vi "ADCP过程数据编码.vi"() -> (3 "发送的信息":string)   [LabVIEW 2016, in "数据传输系统-03.lvlib"]
panel:
  out "数值":i32
  out "层数":string
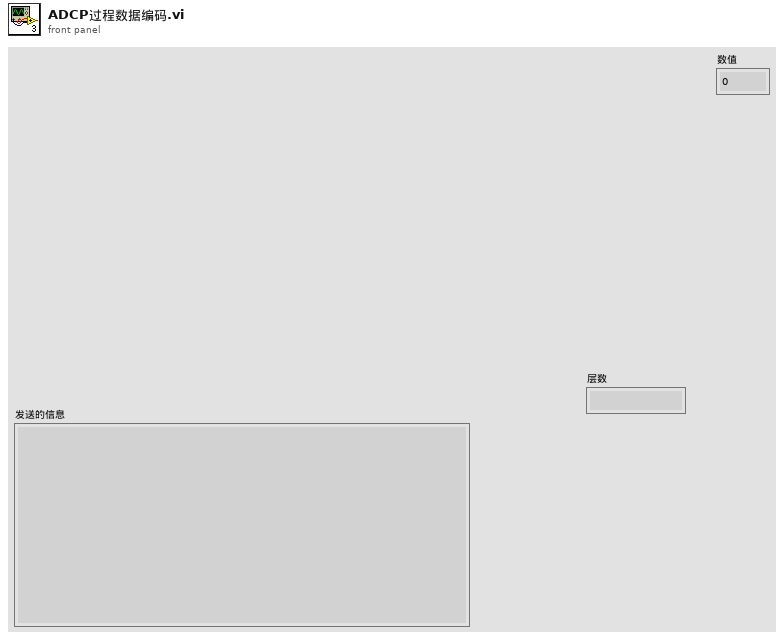
[diagram p1: front panel]
types:
  T1 = cluster{"CODMn":string, "CODCr":string, "DO":string, "铜":string, "PH":string, "氨氮":string, "比电导率":string, "水温":string, "COD":string, "浊度":string, "总氮":string, "总磷":string, "叶绿素a":string, "藻密度":string, "水位":string, "流速":string, "方向":string, "瞬时流量":string, "累积流量":string, "正累积流量":string, "负累积流量":string, "亚硝酸盐":string, "硫化物":string, "ORP":string, "铅":string, "镉":string, "锌":string, "镍":string, "锰":string, "汞":string, "气温":string, "气压":string, "风速":string, "风向":string, "空气温度":string, "相对湿度":string, "分钟雨量":string, "小时雨量":string, "日雨量":string, "累积雨量":string, "盐度":string, "磷酸盐":string, "硝氮":string, "氟化物":string, "挥发酚":string, "氯化物":string, "蓝绿藻":string, "余氯":string, "综合生物毒性":string, "艏向":string, "横摇":string, "纵摇":string, "分层标志":string, "层状态1":string, "层状态2":string, "水平平均流速":string, "流向":string, "北向流速分量":string, "东向流速分量":string, "垂直流速分量":string, "最大波高":string, "最大波周期":string, "1/10波高":string, "1/10波周期":string, "有效波高":string, "有效波周期":string, "平均波高":string, "平均波周期":string, "波向":string, "波个数":string, "水深":string, "X轴流速":string, "Y轴流速":string, "信号强度":string, "电压":string, "悬浮物":string}
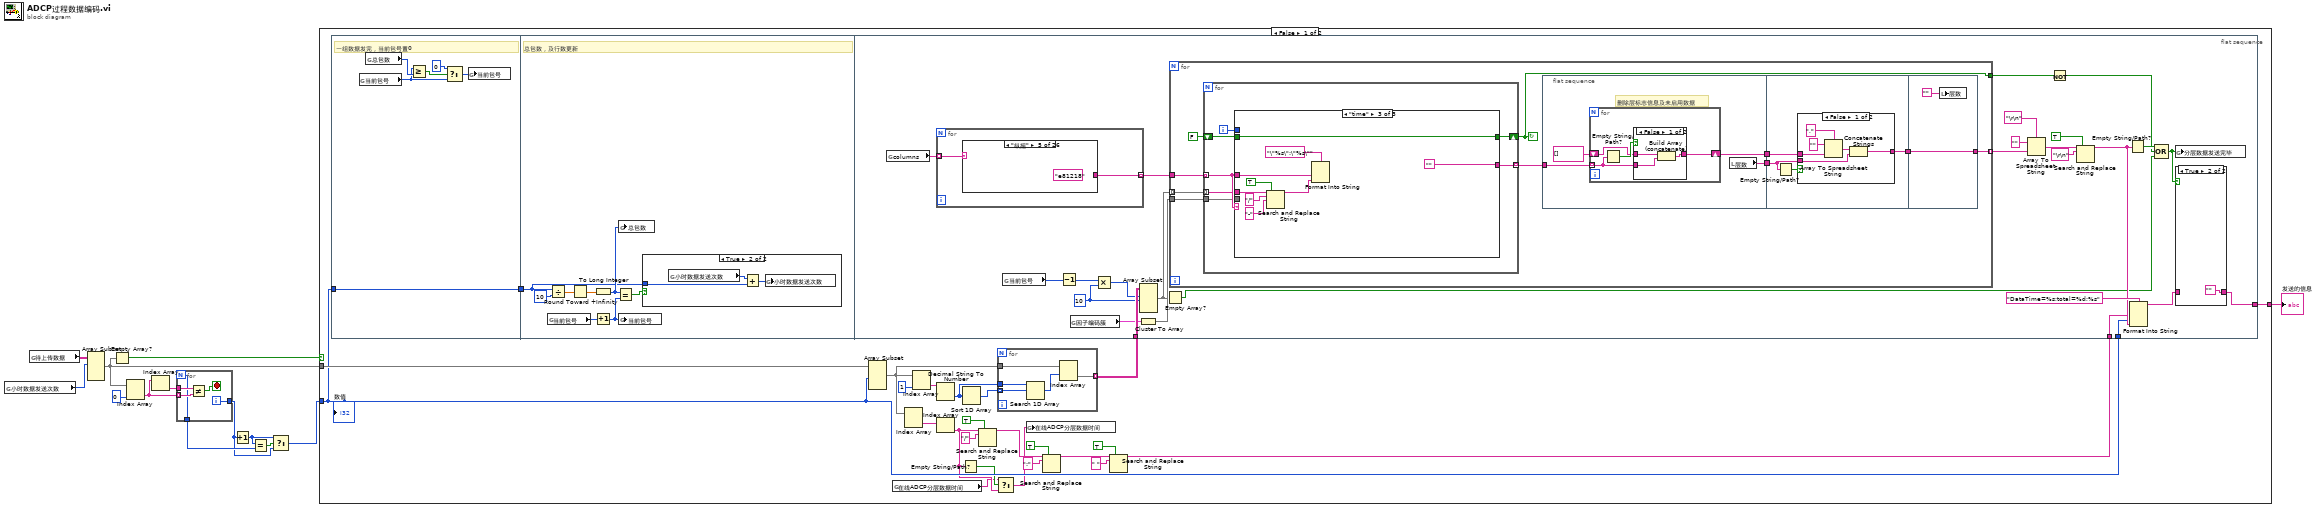
[diagram p0: block diagram]
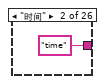
[diagram p5: hidden frame]
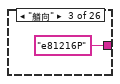
[diagram p6: hidden frame]
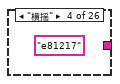
[diagram p7: hidden frame]
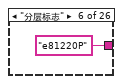
[diagram p8: hidden frame]
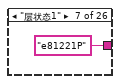
[diagram p9: hidden frame]
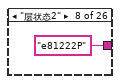
[diagram p10: hidden frame]
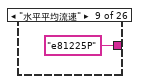
[diagram p11: hidden frame]
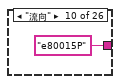
[diagram p12: hidden frame]
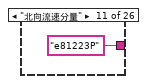
[diagram p13: hidden frame]
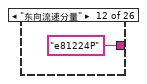
[diagram p14: hidden frame]
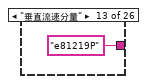
[diagram p15: hidden frame]
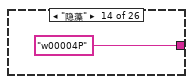
[diagram p16: hidden frame]
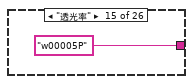
[diagram p17: hidden frame]
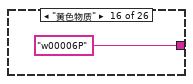
[diagram p18: hidden frame]
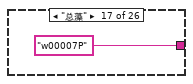
[diagram p19: hidden frame]
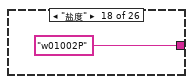
[diagram p20: hidden frame]
diagram:
  n1 = global read "全局 小时数据发送次数.vi" "小时数据发送次数"() -> (w6:i32)
  n2 = global read "全局 所有参数.vi" "待上传数据"() -> (w9:string[][])
  n3 = Array Subset(array=w9, index (row)=w6) -> (w7:string[][])  [unwired: 3 in]
  n4 = Empty Array?(array=w7) -> (empty?=w8:bool)
  n5 = Index Array(array=w7, index (col)=0 ("禁用的索引 (列)")) -> (element=w12:string[])  [unwired: 1 in]
  n6 = Index Array(array=w12) -> (element=w11:string)  [unwired: 1 in]
  n7 = for {
    N -> [w14]
    tunnel: w12 -> [w17] mode=indexing
    tunnel: w11 -> [w18]
    tunnel: [w15] -> w2
    tunnel: [w14] -> w5
    i -> [w15]
    stop <- w16 stop-if-true
    n8 = Not Equal?(x=w18, y=w17) -> (x != y?=w16:bool)
  }
  n9 = Increment(x=w2) -> (x+1=w3:i32)
  n10 = Equal?(x=w3, y=w5) -> (x = y?=w4:bool)
  n11 = Select(t=w3, s=w4, f=w2) -> (s? t:f=w1:i32)
  n12 = case shown="False" w8 {
    selector: w8 -> [_ w198]
    tunnel: w1 -> [w35 _]
    tunnel: w7 -> [w41 _]
    tunnel: [w19 _] -> w10
    frame False {
      n13 = flat-sequence {
        tunnel: w35 -> [w48]
        tunnel: [w48] -> w42
        tunnel: w42 -> [w54]
        tunnel: w37 -> [w91]
        tunnel: w35 -> [w76]
        tunnel: w20 -> [w75]
        tunnel: [w72] -> w19
        frame #0 {
          # "一组数据发完，当前包号置0"
          n14 = global read "全局 数据数组大小.vi" "当前包号"() -> (w51:i32)
          n15 = global read "全局 数据数组大小.vi" "总包数"() -> (w53:i32)
          n16 = Greater Or Equal?(x=w51, y=w53) -> (x >= y?=w52:bool)
          n17 = Select(t=0, s=w52, f=w51) -> (s? t:f=w49:i32)
          n18 = global write "全局 数据数组大小.vi" "当前包号"(w49) -> ()
        }
        frame #1 {
          # "总包数，及行数更新"
          n19 = global read "全局 数据数组大小.vi" "当前包号"() -> (w58:i32)
          n20 = Divide(x=w54, y=10) -> (x/y=w60:dbl)
          n21 = Round Toward +Infinity(x=w60) -> (ceil(x): smallest int >= x=w61:dbl)
          n22 = To Long Integer(number=w61) -> (32bit integer=w57:i32)
          n23 = Increment(x=w58) -> (x+1=w56:i32)
          n24 = Equal?(x=w57, y=w56) -> (x = y?=w55:bool)
          n25 = global write "全局 数据数组大小.vi" "总包数"(w57) -> ()
          n26 = global write "全局 数据数组大小.vi" "当前包号"(w56) -> ()
          n27 = case shown="True" w55 {
            tunnel: w54 -> [_ w63]
            frame False {
            }
            frame True {
              n28 = global read "全局 小时数据发送次数.vi" "小时数据发送次数"() -> (w64:i32)
              n29 = Add(x=w64, y=w63) -> (x+y=w62:i32)
              n30 = global write "全局 小时数据发送次数.vi" "小时数据发送次数"(w62) -> ()
            }
          }
        }
        frame #2 {
          w88 = 10 ("长度")
          n31 = global read "全局 所有参数.vi" "columns"() -> (w85:string[])
          n32 = for {
            tunnel: w85 -> [w95] mode=indexing
            tunnel: [w94] -> w84 mode=indexing
            n33 = case shown="\"纵摇\"" w95 {
              tunnel: [_ "time" ("元素") "e81216P" _ _ "e81220P" "e81221P" "e81222P" "e81225P" "e80015P" "e81223P" "e81224P" "e81219P" "w00004P" "w00005P" "w00006P" "w00007P" "w01002P" "w01022P" "w81024P" "w81025P" "w81023P" "e81226" "e81227" "row" ("元素") "e81228"] -> w94
              frame "", Default {
              }
              frame "时间" {
              }
              frame "艏向" {
              }
              frame "横摇" {
                (unwired) "e81217"
              }
              frame "纵摇" {
                (unwired) "e81218"
              }
              frame "分层标志" {
              }
              frame "层状态1" {
              }
              frame "层状态2" {
              }
              frame "水平平均流速" {
              }
              frame "流向" {
              }
              frame "北向流速分量" {
              }
              frame "东向流速分量" {
              }
              frame "垂直流速分量" {
              }
              frame "隐藻" {
              }
              frame "透光率" {
              }
              frame "黄色物质" {
              }
              frame "总藻" {
              }
              frame "盐度" {
              }
              frame "蓝绿藻" {
              }
              frame "Fv/Fm" {
              }
              frame "PAR" {
              }
              frame "GPP" {
              }
              frame "X轴流速" {
              }
              frame "Y轴流速" {
              }
              frame "层数" {
              }
              frame "信号强度" {
              }
            }
          }
          n34 = global read "全局 数据数组大小.vi" "当前包号"() -> (w90:i32)
          n35 = Decrement(x=w90) -> (x-1=w89:i32)
          n36 = global read "断电保存全局.vi" "因子编码簇"() -> (w87:T1)
          n37 = Multiply(x=w89, y=w88) -> (x*y=w83:i32)
          n38 = Array Subset(array=w91, index (row)=w83, length (row)=w88) -> (w71:string[][])  [unwired: 2 in]
          n39 = Cluster To Array(cluster=w87) -> (array=w86:string[])
          n40 = Empty Array?(array=w71) -> (empty?=w68:bool)
          n41 = for {
            tunnel: w71 -> [w127] mode=indexing
            tunnel: w84 -> [w128]
            tunnel: [w120] -> w77 mode=indexing
            tunnel: w86 -> [w125]
            tunnel: [w123] -> w74
            stop <- w123 continue-if-true
            n42 = for {
              tunnel: w128 -> [w159] mode=indexing
              tunnel: w127 -> [w158] mode=indexing
              tunnel: [w160] -> w126 mode=indexing
              tunnel: w125 -> [w156]
              shift-right: [w154] -> w123
              shift-left: FALSE -> [w155]
              i -> [w157]
              n43 = case shown="\"time\"" w159 {
                selector: w159 -> [w165 _ _]
                tunnel: [w175 "" ""] -> w160
                tunnel: w159 -> [w174 w187 w196]
                tunnel: w158 -> [w173 w186 w192]
                tunnel: w157 -> [_ _ _]
                tunnel: w156 -> [w172 _ _]
                tunnel: w155 -> [w168 w184 w190]
                tunnel: [w169 w184 w190] -> w154
                frame "", Default {
                  n44 = String Subset(string=w165, length (rest)=6 ("长度（剩余）")) -> (substring=w166:string)  [unwired: 1 in]
                  n45 = global read "断电保存全局.vi" "参数启用数组"() -> (w171:bool[])
                  n46 = Search 1D Array(1D array=w172, element=w166) -> (index of element=w170:i32)  [unwired: 1 in]
                  n47 = Empty String/Path?(string/path=w165) -> (empty?=w164:bool)
                  n48 = Not(x=w164) -> (.not. x?=w163:bool)
                  n49 = Index Array(array=w171, index=w170) -> (element=w162:bool)
                  n50 = And(x=w162, y=w163) -> (x .and. y?=w161:bool)
                  n51 = case shown="True" w161 {
                    tunnel: ["" w181] -> w175
                    tunnel: w174 -> [_ w180]
                    tunnel: w173 -> [_ w179]
                    tunnel: [w176 TRUE] -> w169
                    tunnel: w168 -> [w176 _]
                    frame False {
                    }
                    frame True {
                      n52 = Format Into String(format string="%s-Rtd=%s" ("格式字符串"), w180, w179) -> (resulting string=w181:string)  [unwired: 2 in, 1 out]
                    }
                  }
                }
                frame "row" {
                  n53 = Format Into String(format string=",%s=%s;" ("格式字符串"), w187, w186) -> (resulting string=→"层数":string)  [unwired: 2 in, 1 out]
                }
                frame "time" {
                  n54 = Search and Replace String(replace all?=TRUE ("替换全部？(F)"), input string=w192, search string="/" ("搜索字符串"), replace string="-" ("替换字符串(\"\")")) -> (result string=w191:string)  [unwired: 4 in, 3 out]
                  n55 = Format Into String(format string="\"%s\":\"%s\"" ("格式字符串"), w196, w191) -> ()  [unwired: 2 in, 2 out]
                }
              }
            }
            n56 = flat-sequence {
              tunnel: w126 -> [w131]
              tunnel: [w132] -> w122
              tunnel: [w129] -> w121
              tunnel: w122 -> [w142]
              tunnel: w121 -> [w144]
              tunnel: [w141] -> w119
              tunnel: [w153] -> w120
              tunnel: w119 -> [w153]
              frame #0 {
                # "删除层标志信息及未启用数据"
                n57 = for {
                  tunnel: w131 -> [w133] mode=indexing
                  shift-right: [w134] -> w129
                  shift-left: string[] [] -> [w135]
                  n58 = Empty String/Path?(string/path=w133) -> (empty?=w136:bool)
                  n59 = case shown="False" w136 {
                    tunnel: [w137 w140] -> w134
                    tunnel: w135 -> [w139 w140]
                    tunnel: w133 -> [w138 _]
                    frame False {
                      n60 = Build Array (concatenate)(w139, w138) -> (w137:string[])
                    }
                    frame True {
                    }
                  }
                }
                n61 = local read "层数"() -> (w132:string)
              }
              frame #1 {
                n62 = Empty String/Path?(string/path=w142) -> (empty?=w143:bool)
                n63 = case shown="False" w143 {
                  tunnel: w144 -> [w147 _]
                  tunnel: w142 -> [w146 _]
                  tunnel: [w145 ""] -> w141
                  frame False {
                    n64 = Array To Spreadsheet String(delimiter (Tab)="," ("分隔符(Tab)"), array=w147, 3:"" ("格式字符串")) -> (spreadsheet string=w150:string)
                    n65 = Concatenate Strings(w150, w146) -> (w145:string)
                  }
                  frame True {
                  }
                }
              }
              frame #2 {
                n66 = local write "层数"("") -> ()
              }
            }
          }
          n67 = Array To Spreadsheet String(delimiter (Tab)="\r\n", array=w77, 3:"" ("格式字符串")) -> (spreadsheet string=w67:string)
          n68 = Not(x=w74) -> (.not. x?=w69:bool)
          n69 = Search and Replace String(replace all?=TRUE ("替换全部？(F)"), input string=w67, search string="\r\n") -> (result string=w78:string)  [unwired: 5 in, 3 out]
          n70 = Empty String/Path?(string/path=w78) -> (empty?=w70:bool)
          n71 = Format Into String(format string="DataTime=%s;total=%d;%s", w75, w76, w78) -> (resulting string=w73:string)  [unwired: 2 in, 1 out]
          n72 = Compound Arithmetic op=OR ("复合运算")(w70, w69, w68) -> (w66:bool)
          n73 = global write "全局 数据数组大小.vi" "分层数据发送完毕"(w66) -> ()
          n74 = case shown="True" w66 {
            tunnel: [w92 ""] -> w72
            tunnel: w73 -> [w92 _]
            frame False {
            }
            frame True {
            }
          }
        }
      }
      n75 = Array Subset(array=w41, length (row)=w35) -> (w21:string[][])  [unwired: 3 in]
      n76 = global read "全局 水样时间.vi" "在线ADCP分层数据时间"() -> (w23:string)
      n77 = Index Array(array=w21) -> (element=w34:string[])  [unwired: 2 in]
      n78 = Index Array(array=w21, index (col)=1 ("禁用的索引 (列)")) -> (element=w40:string[])  [unwired: 1 in]
      n79 = Decimal String To Number(string=w40) -> (number=w39:i32[])  [unwired: 2 in, 1 out]
      n80 = Index Array(array=w34) -> (element=w24:string)  [unwired: 1 in]
      n81 = Empty String/Path?(string/path=w24) -> (empty?=w25:bool)
      n82 = Sort 1D Array(array=w39) -> (sorted array=w38:i32[])
      n83 = Search and Replace String(replace all?=TRUE ("替换全部？(F)"), input string=w24, search string="/" ("替换字符串(\"\")")) -> (result string=w29:string)  [unwired: 5 in, 3 out]
      n84 = Select(t=w23, s=w25, f=w24) -> (s? t:f=w22:string)
      n85 = for {
        tunnel: w39 -> [w47]
        tunnel: w38 -> [w46] mode=indexing
        tunnel: w21 -> [w45]
        tunnel: [w43] -> w37 mode=indexing
        n86 = Search 1D Array(1D array=w47, element=w46) -> (index of element=w44:i32)  [unwired: 1 in]
        n87 = Index Array(array=w45, index (row)=w44) -> (element=w43:string[])  [unwired: 1 in]
      }
      n88 = global write "全局 水样时间.vi" "在线ADCP分层数据时间"(w22) -> ()
      n89 = Search and Replace String(replace all?=TRUE ("替换全部？(F)"), input string=w29, search string=":" ("替换字符串(\"\")")) -> (result string=w26:string)  [unwired: 5 in, 3 out]
      n90 = Search and Replace String(replace all?=TRUE ("替换全部？(F)"), input string=w26, search string=" " ("替换字符串(\"\")")) -> (result string=w20:string)  [unwired: 5 in, 3 out]
      "数值" <- w35
    }
    frame True {
      n91 = global write "全局 数据数组大小.vi" "分层数据发送完毕"(w198) -> ()
    }
  }
  "发送的信息" <- w10
